vi "Teleop.vi"(10 "Match Info":T2={"Autonomous Elapsed Seconds"=0.0, "TeleOp Elapsed Seconds"=18.704, "Disabled Elapsed Seconds"=49.24, "Visited Autonomous"=FALSE, "Visited TeleOp"=TRUE, "Visited Disabled"=TRUE, "Autonomous Settings"={"Autonomous Style"=enum."Independent", "VI Refnum"=refnum}}, 11 "Call Context":T3=enum."Execute") -> ()   [LabVIEW 2015]
doc: "This VI is called for each TeleOp packet received from the DS where the robot is not disabled. It is often used to read from the joysticks and update I/O or to update setpoints for timed control loops. It should complete and return within 20 milliseconds or it may miss DS packets."
uses:
  <vilib>/Rock Robotics/WPI/DriverStation/WPI_DriverStationDerivedRobotMode.ctl
  <vilib>/Rock Robotics/WPI/DriverStation/WPI_DriverStationMatch Info.ctl
  shooter/shooter.lvclass/shooter.ctl
  intake/intake.lvclass/intake.ctl
  <vilib>/Rock Robotics/Network Tables/NT Read Boolean.vi
  <vilib>/Rock Robotics/Network Tables/NT Read Number.vi
  <vilib>/Rock Robotics/WPI/Utilities/WPI_GetSetVariantRefNum.vi
  Robot Global Data.vi
  <vilib>/Rock Robotics/Network Tables/NT Write Boolean.vi
  <vilib>/Rock Robotics/WPI/RobotDrive/WPI_RobotDriveArcadeDrive_Standard(NoSaturation).vi
  <vilib>/addons/control/pid/pid.llb/PID (DBL).vi
  <vilib>/Rock Robotics/Network Tables/NT Write Number.vi
  <vilib>/addons/control/pid/NI_PID_pid.lvlib
  <vilib>/addons/control/pid/pid.llb/PID Output Rate Limiter (DBL).vi
  shooter/shooter.lvclass
  intake/intake.lvclass
panel:
  out "Waveform Chart":cluster{dbl, dbl}(graph)={-0.002641071322889855, -0.1}
  in  "PID gains":T1={"proportional gain (Kc)"=1.0, "integral time (Ti, min)"=0.01, "derivative time (Td, min)"=0.0} {"derivative time (Td, min)" format="%.3f"; "integral time (Ti, min)" format="%.3f"; "proportional gain (Kc)" format="%.3f"}
  out "Sample Slider 0":dbl(slide) scale=0.0..5.0
  out "Sample Boolean 0":bool
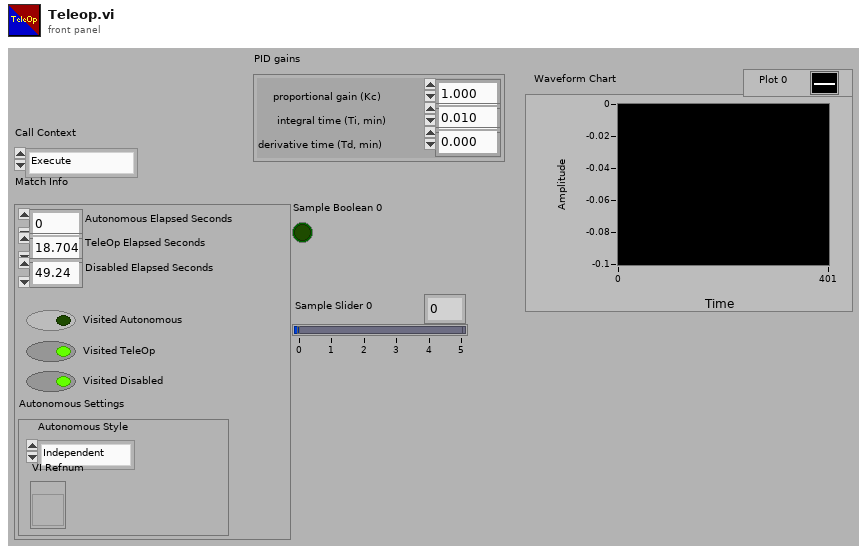
[diagram p1: front panel]
types:
  T1 = cluster{"proportional gain (Kc)":dbl, "integral time (Ti, min)":dbl, "derivative time (Td, min)":dbl}
  T2 = typedef "WPI_DriverStationMatch Info.ctl" = cluster{"Autonomous Elapsed Seconds":dbl, "TeleOp Elapsed Seconds":dbl, "Disabled Elapsed Seconds":dbl, "Visited Autonomous":bool, "Visited TeleOp":bool, "Visited Disabled":bool, "Autonomous Settings":cluster{"Autonomous Style":enum16{"Iterative", "Independent"}, "VI Refnum":refnum<vi>}}
  T3 = typedef "WPI_DriverStationDerivedRobotMode.ctl" = enum16{"Init", "Execute", "Stop"}
  T4 = typedef "WPI_JoystickDevRef.ctl" = cluster{"Device":T5}
  T5 = typedef "WPI_JoystickDeviceEnum.ctl" = enum16{"USB 0", "USB 1", "USB 2", "USB 3", "USB 4", "USB 5"}
  T6 = typedef "WPI_MotorControlDeviceRef.ctl" = cluster{"DeviceStatus":errorcluster, "Type":T7, "PWM":cluster{"PWM Channel":T8, "DeadBand":T9}, "CAN":cluster{"Device Number":u8, "Control Mode":T10, "Semaphore":T11, "Max Vout":dbl, "TalonSRX Control Mode":T12}, "Invert":bool}
  T7 = typedef "WPI_MotorControlType.ctl" = enum16{"PWM", "CAN", "CANTalonSRX"}
  T8 = typedef "FPGA_DIOPWMChannel.ctl" = enum8{"PWM 0", "PWM 1", "PWM 2", "PWM 3", "PWM 4", "PWM 5", "PWM 6", "PWM 7", "PWM 8", "PWM 9", "PWM MXP 0", "PWM MXP 1", "PWM MXP 2", "PWM MXP 3", "PWM MXP 4", "PWM MXP 5", "PWM MXP 6", "PWM MXP 7", "PWM MXP 8", "PWM MXP 9", "Invalid"}
  T9 = typedef "WPI_PWMDeadband.ctl" = cluster{"Name":string, "maxPositivePwm":i32, "minPositivePwm":i32, "centerPwm":i32, "maxNegativePwm":i32, "minNegativePwm":i32, "angularRange":u16}
  T10 = typedef "WPI_CANJaguar_ControlMode.ctl" = enum8{"Percent VBus", "Current", "Speed", "Position", "Voltage"}
  T11 = typedef "Semaphore RefNum" = refnum<k1>
  T12 = typedef "WPI_CANTalonSRX_APIControlMode.ctl" = enum8{"Percent VBus", "Speed", "Position", "Slave", "Unchanged / Invalid", "Voltage Compensation", "Current", "Motion Profile"}
  T13 = typedef "WPI_RobotDriveDevRef.ctl" = cluster{"DevStatus":errorcluster, "Motors[]":T6[], "Square Inputs":bool, "Max Output":dbl}
  T14 = typedef "WPI_SwitchDevRef.ctl" = cluster{"DevStatus":errorcluster, "DIO Channel":T15, "CntIndex":T16, "Normally Closed":bool}
  T15 = typedef "FPGA_DIOChannel.ctl" = enum8{"DIO 0", "DIO 1", "DIO 2", "DIO 3", "DIO 4", "DIO 5", "DIO 6", "DIO 7", "DIO 8", "DIO 9", "DIO MXP 0", "DIO MXP 1", "DIO MXP 2", "DIO MXP 3", "DIO MXP 4", "DIO MXP 5", "DIO MXP 6", "DIO MXP 7", "DIO MXP 8", "DIO MXP 9", "DIO MXP 10", "DIO MXP 11", "DIO MXP 12", "DIO MXP 13", "DIO MXP 14", "DIO MXP 15", "Invalid"}
  T16 = typedef "FPGA_CounterCtrSystemIndex.ctl" = enum8{"Ctr 0", "Ctr 1", "Ctr 2", "Ctr 3", "Ctr 4", "Ctr 5", "Ctr 6", "Ctr 7", "Invalid"}
  T17 = typedef "WPI_PotentiometerDevRef.ctl" = cluster{"DevStatus":errorcluster, "Analog Channel":T18, "Invert Output":bool}
  T18 = typedef "FPGA_AIChannel.ctl" = enum8{"AI 0", "AI 1", "AI 2", "AI 3", "AI MXP 0", "AI MXP 1", "AI MXP 2", "AI MXP 3", "Invalid"}
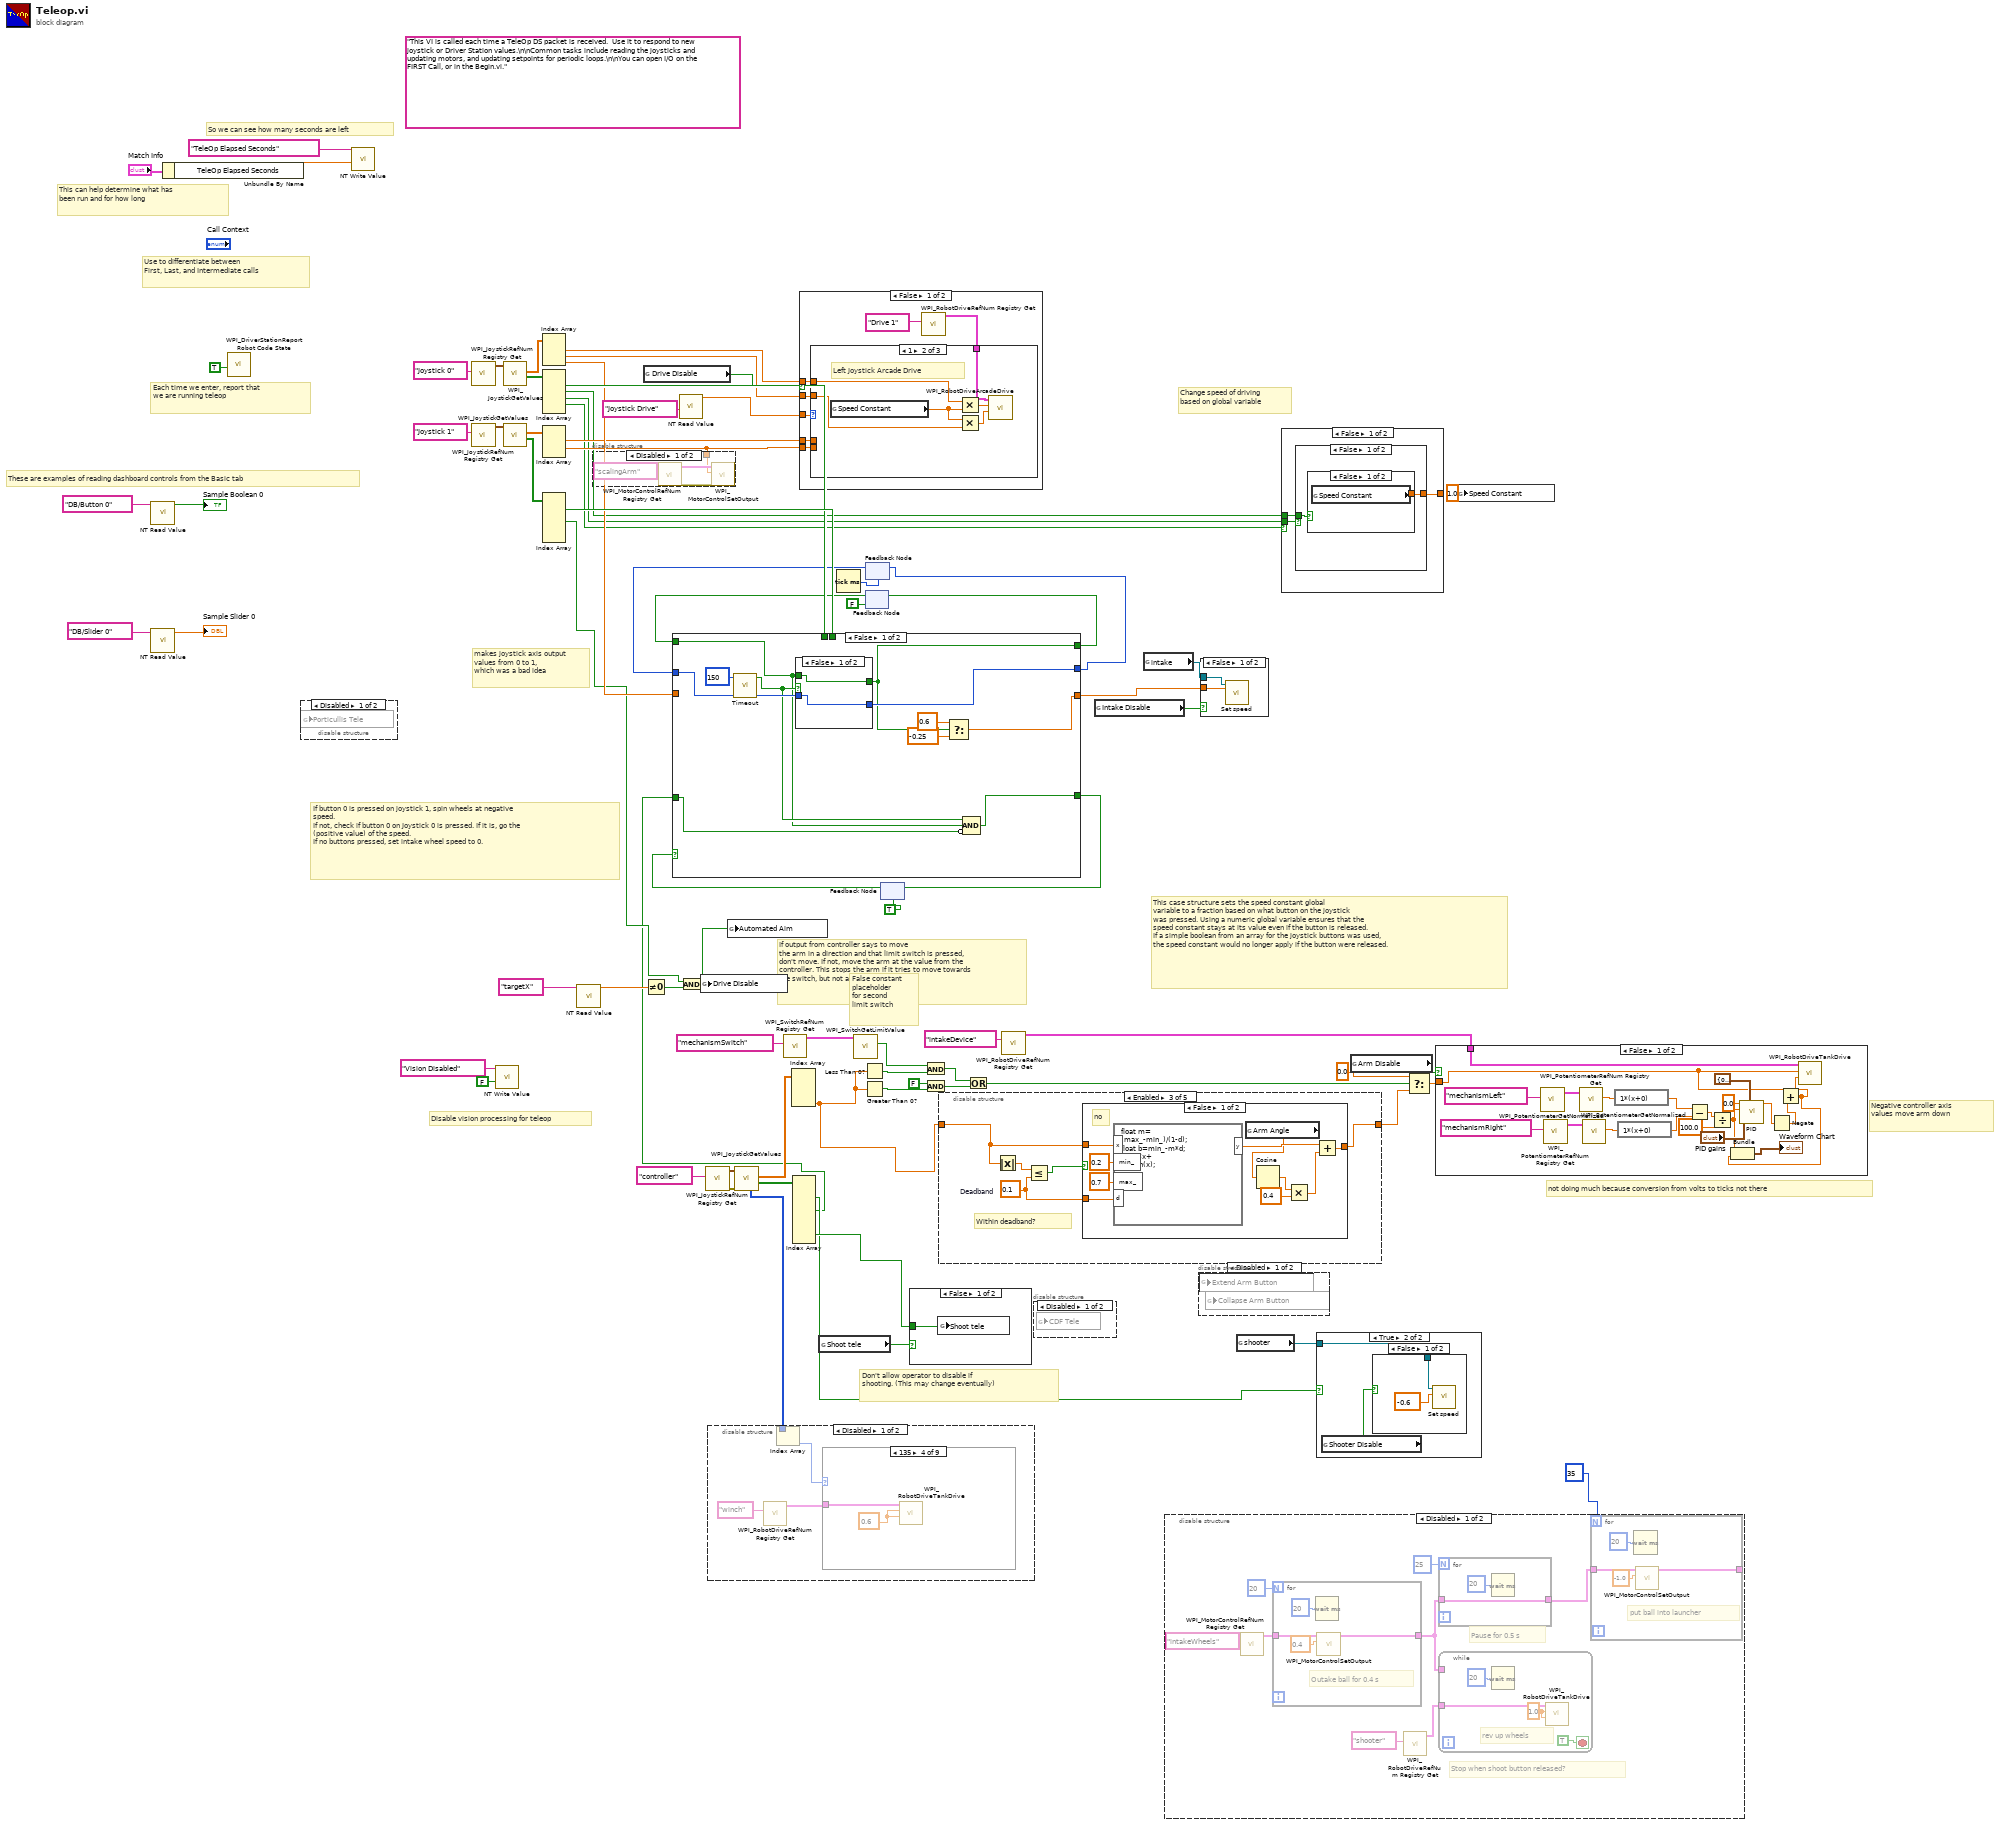
[diagram p0: block diagram]
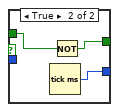
[diagram p4: hidden frame]
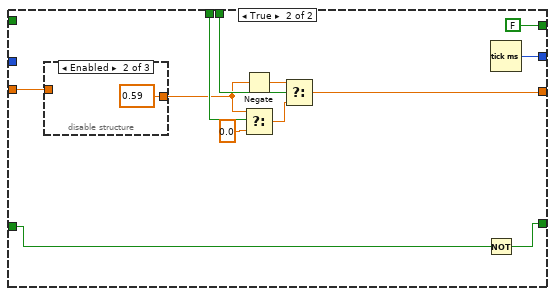
[diagram p5: hidden frame]
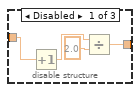
[diagram p6: hidden frame]
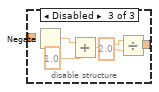
[diagram p7: hidden frame]
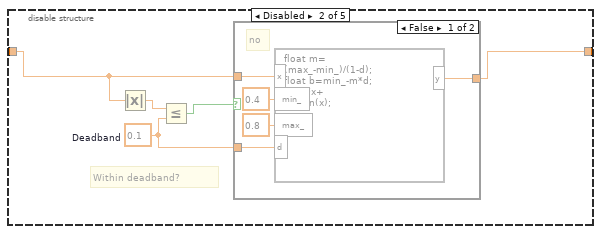
[diagram p13: hidden frame]
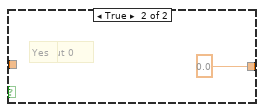
[diagram p14: hidden frame]
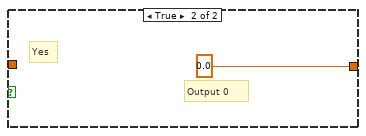
[diagram p15: hidden frame]
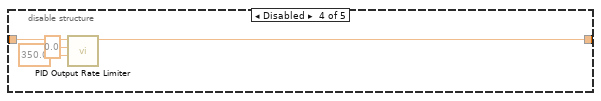
[diagram p16: hidden frame]
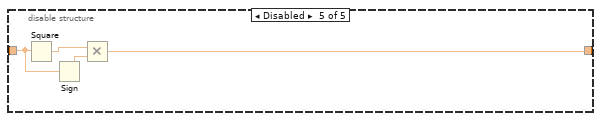
[diagram p17: hidden frame]
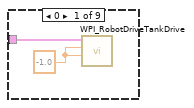
[diagram p18: hidden frame]
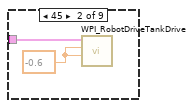
[diagram p19: hidden frame]
diagram:
  (unwired) "This VI is called each time a TeleOp DS packet is received.  Use it to respond to new joystick or Driver Station values.\n\nCommon tasks include reading the joysticks and updating motors, and updating setpoints for periodic loops.\n\nYou can open I/O on the FIRST Call, or in the Begin.vi."
  # "Don't allow operator to disable if\nshooting. (This may change eventually)"
  # "not doing much because conversion from volts to ticks not there"
  # "So we can see how many seconds are left"
  # "makes joystick axis output\nvalues from 0 to 1,\nwhich was a bad idea"
  # "If output from controller says to move \nthe arm in a direction and that limit switch is pressed,\ndon't move. If not, move the arm at the value from the\ncontroller. This stops the arm if it tries to move towards\nthe switch, but not away."
  # "False constant \nplaceholder\nfor second \nlimit switch"
  # "Disable vision processing for teleop"
  # "Change speed of driving\nbased on global variable"
  # "If button 0 is pressed on joystick 1, spin wheels at negative\nspeed.\nIf not, check if button 0 on Joystick 0 is pressed. If it is, go the\n(positive value) of the speed.\nIf no buttons pressed, set intake wheel speed to 0."
  # "Negative controller axis\nvalues move arm down"
  # "This case structure sets the speed constant global\nvariable to a fraction based on what button on the joystick\nwas pressed. Using a numeric global variable ensures that the\nspeed constant stays at its value even if the button is released.\nIf a simple boolean from an array for the joystick buttons was used,\nthe speed constant would no longer apply if the button were released."
  # "These are examples of reading dashboard controls from the Basic tab"
  # "Each time we enter, report that\nwe are running teleop"
  # "Use to differentiate between\nFirst, Last, and Intermediate calls"
  # "This can help determine what has\nbeen run and for how long"
  n1 = call-poly <vilib>:"NT Read Value.vi"("Name"="DB/Button 0" ("refnum name")) -> ("Boolean"=→"Sample Boolean 0":bool)  [unwired: 9 in, 1 out]
  n2 = call-poly <vilib>:"NT Read Value.vi"("Name"="DB/Slider 0" ("refnum name")) -> ("Numeric"=→"Sample Slider 0":dbl)  [unwired: 9 in, 1 out]
  n3 = Unbundle By Name("Match Info") -> ("TeleOp Elapsed Seconds"=w60:dbl)
  n4 = call <vilib>:"WPI_DriverStationReport Robot Code State.vi"("TeleOp"=TRUE ("Autonomous")) -> ()  [unwired: 10 in, 1 out]
  n5 = disable-structure shown="Disabled" {
    frame Disabled {
      n6 = global read "Robot Global Data.vi" "Porticullis Tele"() -> ()  [unwired: 1 in]
    }
    frame Enabled {
    }
  }
  n7 = call-poly <vilib>:"NT Write Value.vi"("Numeric"=w60, "Name"="TeleOp Elapsed Seconds") -> ()  [unwired: 9 in, 1 out]
  n8 = call <vilib>:"WPI_JoystickRefNum Registry Get.vi"("refnum name"="Joystick 0") -> ("JoystickDevRef"=w57:T4)  [unwired: 9 in, 1 out]
  n9 = call <vilib>:"WPI_JoystickRefNum Registry Get.vi"("refnum name"="Joystick 1") -> ("JoystickDevRef"=w54:T4)  [unwired: 9 in, 1 out]
  n10 = call-poly <vilib>:"NT Write Value.vi"("Boolean"=FALSE, "Name"="Vision Disabled") -> ()  [unwired: 9 in, 1 out]
  n11 = call <vilib>:"WPI_JoystickGetValues.vi"("JoystickDevRef"=w57) -> ("Buttons"=w41:bool[], "Axes"=w56:dbl[])  [unwired: 6 in, 3 out]
  n12 = call <vilib>:"WPI_JoystickGetValues.vi"("JoystickDevRef"=w54) -> ("Buttons"=w52:bool[], "Axes"=w53:dbl[])  [unwired: 6 in, 3 out]
  n13 = Index Array(array=w56) -> (element #1=w36:dbl, element #2=w39:dbl, element #3=w45:dbl)  [unwired: 3 in]
  n14 = Index Array(array=w41) -> (element #1=w50:bool, element #2=w22:bool, element #3=w6:bool, element #4=w21:bool)  [unwired: 5 in, 1 out]
  n15 = Index Array(array=w53) -> (element #1=w35:dbl, element #2=w32:dbl)  [unwired: 3 in, 1 out]
  n16 = Index Array(array=w52) -> (element #1=w51:bool, element #3=w17:bool)  [unwired: 6 in, 4 out]
  n17 = call-poly <vilib>:"NT Read Value.vi"("Name"="targetX") -> ("Numeric"=w19:dbl)  [unwired: 9 in, 1 out]
  n18 = disable-structure shown="Disabled" {
    disable-tunnel: w32 -> [w78 _]
    frame Disabled {
      n19 = call <vilib>:"WPI_MotorControlRefNum Registry Get.vi"("refnum name"="scalingArm") -> ("error out"=w80:errorcluster, "MotorControlDevRef"=w81:T6)  [unwired: 9 in]
      n20 = call <vilib>:"WPI_MotorControlSetOutput.vi"("error in (no error)"=w80, "Output"=w78, "MotorControlDevRef"=w81) -> ()  [unwired: 6 in, 3 out]
    }
    frame Enabled {
    }
  }
  n21 = global read "Robot Global Data.vi" "Drive Disable"() -> (w34:bool)
  n22 = Not Equal To 0?(x=w19) -> (x != 0?=w18:bool)
  n23 = call-poly <vilib>:"NT Read Value.vi"("Name"="Joystick Drive") -> ("Numeric"=w37:dbl)  [unwired: 9 in, 1 out]
  n24 = And(x=w17, y=w18) -> (x .and. y?=w16:bool)
  n25 = global write "Robot Global Data.vi" "Drive Disable"(w16) -> ()
  n26 = call <vilib>:"WPI_JoystickRefNum Registry Get.vi"("refnum name"="controller") -> ("error out"=w70:errorcluster, "JoystickDevRef"=w69:T4)  [unwired: 9 in]
  n27 = global write "Robot Global Data.vi" "Automated Aim"(w16) -> ()
  n28 = call <vilib>:"WPI_JoystickGetValues.vi"("error in (no error)"=w70, "JoystickDevRef"=w69) -> ("Buttons"=w71:bool[], "Axes"=w67:dbl[], "POVs"=w33:i16[])  [unwired: 5 in, 2 out]
  n29 = disable-structure shown="Disabled" {
    disable-tunnel: w33 -> [w85 _]
    frame Disabled {
      n30 = call <vilib>:"WPI_RobotDriveRefNum Registry Get.vi"("refnum name"="winch") -> ("RobotDriveDevRef"=w82:T13)  [unwired: 9 in, 1 out]
      n31 = Index Array(array=w85) -> (element=w84:i16)  [unwired: 1 in]
      n32 = case shown="135" w84 {
        tunnel: w82 -> [w87 w89 _ w90 w93 w94 _ w96 _]
        frame 0 {
          w86 = -1.0 ("Left axis value")
          n33 = call <vilib>:"WPI_RobotDriveTankDrive.vi"("Right axis value"=w86, "Left axis value"=w86, "RobotDriveDevRef"=w87) -> ()  [unwired: 6 in, 3 out]
        }
        frame 45 {
          w88 = -0.6 ("Left axis value")
          n34 = call <vilib>:"WPI_RobotDriveTankDrive.vi"("Right axis value"=w88, "Left axis value"=w88, "RobotDriveDevRef"=w89) -> ()  [unwired: 6 in, 3 out]
        }
        frame 90 {
        }
        frame 135 {
          w91 = 0.6 ("Left axis value")
          n35 = call <vilib>:"WPI_RobotDriveTankDrive.vi"("Right axis value"=w91, "Left axis value"=w91, "RobotDriveDevRef"=w90) -> ()  [unwired: 6 in, 3 out]
        }
        frame 180 {
          w92 = 1.0 ("Left axis value")
          n36 = call <vilib>:"WPI_RobotDriveTankDrive.vi"("Right axis value"=w92, "Left axis value"=w92, "RobotDriveDevRef"=w93) -> ()  [unwired: 6 in, 3 out]
        }
        frame 225 {
          w95 = -0.6 ("Left axis value")
          n37 = call <vilib>:"WPI_RobotDriveTankDrive.vi"("Right axis value"=w95, "Left axis value"=w95, "RobotDriveDevRef"=w94) -> ()  [unwired: 6 in, 3 out]
        }
        frame 270 {
        }
        frame 315 {
          w97 = -1.0 ("Left axis value")
          n38 = call <vilib>:"WPI_RobotDriveTankDrive.vi"("Right axis value"=w97, "Left axis value"=w97, "RobotDriveDevRef"=w96) -> ()  [unwired: 6 in, 3 out]
        }
        frame -1, Default {
        }
      }
    }
    frame Enabled {
    }
  }
  n39 = call <vilib>:"WPI_SwitchRefNum Registry Get.vi"("refnum name"="mechanismSwitch") -> ("SwitchDevRef"=w63:T14)  [unwired: 9 in, 1 out]
  n40 = Index Array(array=w67) -> (element #4=w23:dbl)  [unwired: 4 in, 3 out]
  n41 = Index Array(array=w71) -> (element #2=w4:bool, element #4=w3:bool, element #8=w28:bool)  [unwired: 9 in, 6 out]
  n42 = case shown="False" w34 {
    tunnel: w39 -> [w103 _]
    tunnel: w32 -> [w102 _]
    tunnel: w37 -> [w100 _]
    tunnel: w36 -> [w99 _]
    tunnel: w35 -> [w98 _]
    frame False {
      n43 = call <vilib>:"WPI_RobotDriveRefNum Registry Get.vi"("refnum name"="Drive 1") -> ("RobotDriveDevRef"=w101:T13)  [unwired: 9 in, 1 out]
      n44 = case shown="1" w100 {
        tunnel: w103 -> [w107 w112 _]
        tunnel: w102 -> [w106 _ w118]
        tunnel: w101 -> [w105 w113 w117]
        tunnel: w99 -> [_ w111 _]
        tunnel: w98 -> [_ _ w119]
        frame 0, Default {
          # "Both Joysticks Tank Drive"
          n45 = global read "Robot Global Data.vi" "Speed Constant"() -> (w108:dbl)
          n46 = Multiply(x=w107, y=w108) -> (x*y=w109:dbl)
          n47 = Multiply(x=w108, y=w106) -> (x*y=w110:dbl)
          n48 = call <vilib>:"WPI_RobotDriveTankDrive.vi"("Right axis value"=w110, "Left axis value"=w109, "RobotDriveDevRef"=w105) -> ()  [unwired: 6 in, 3 out]
        }
        frame 1 {
          # "Left Joystick Arcade Drive"
          n49 = global read "Robot Global Data.vi" "Speed Constant"() -> (w116:dbl)
          n50 = Multiply(x=w111, y=w116) -> (x*y=w115:dbl)
          n51 = Multiply(x=w116, y=w112) -> (x*y=w114:dbl)
          n52 = call-poly <vilib>:"WPI_RobotDriveArcadeDrive.vi"("Y axis value"=w114, "X axis value"=w115, "RobotDriveDevRef"=w113) -> ()  [unwired: 6 in, 3 out]
        }
        frame 2 {
          # "Right Joystick Arcade Drive"
          n53 = global read "Robot Global Data.vi" "Speed Constant"() -> (w122:dbl)
          n54 = Multiply(x=w119, y=w122) -> (x*y=w121:dbl)
          n55 = Multiply(x=w122, y=w118) -> (x*y=w120:dbl)
          n56 = call-poly <vilib>:"WPI_RobotDriveArcadeDrive.vi"("Y axis value"=w120, "X axis value"=w121, "RobotDriveDevRef"=w117) -> ()  [unwired: 6 in, 3 out]
        }
      }
    }
    frame True {
      # "Drive motors are controlled by\nloop in periodic tasks"
    }
  }
  n57 = global read "Robot Global Data.vi" "Shoot tele"() -> (w29:bool)
  n58 = Tick Count (ms)() -> (millisecond timer value=w7:u32)
  n59 = call <vilib>:"WPI_SwitchGetLimitValue.vi"("SwitchDevRef"=w63) -> ("Switch Pressed"=w62:bool)  [unwired: 8 in, 2 out]
  n60 = Less Than 0?(x=w23) -> (x < 0?=w61:bool)
  n61 = Greater Than 0?(x=w23) -> (x > 0?=w49:bool)
  n62 = feedback #1(FALSE ("Intake Disable")) -> (w11:bool)
  n63 = feedback #2(w7) -> (w8:u32)
  n64 = feedback #3(TRUE ("Intake Disable")) -> (w13:bool)
  n65 = case shown="False" w13 {
    tunnel: w51 -> [_ w149]
    tunnel: w50 -> [_ w148]
    tunnel: w45 -> [_ w146]
    tunnel: [w125 w144] -> w26
    tunnel: [w126 FALSE ("Intake Disable")] -> w12
    tunnel: w11 -> [w129 _]
    tunnel: [w131 w142] -> w9
    tunnel: w8 -> [w133 _]
    tunnel: [w127 w140] -> w5
    tunnel: w3 -> [w128 w141]
    frame False {
      n66 = call "Timeout.vi"("Start Time In"=w133, "Time Limit"=u32 150) -> ("Start Time Out"=w132:u32, "Timeout"=w130:bool)  [unwired: 8 in]
      n67 = case shown="False" w130 {
        tunnel: w132 -> [w136 _]
        tunnel: [w136 w139] -> w131
        tunnel: w129 -> [w135 w138]
        tunnel: [w135 w137] -> w126
        frame False {
        }
        frame True {
          n68 = Tick Count (ms)() -> (millisecond timer value=w139:u32)
          n69 = Not(x=w138) -> (.not. x?=w137:bool)
        }
      }
      n70 = Select(t=0.6, s=w126, f=-0.25) -> (s? t:f=w125:dbl)
      n71 = Compound Arithmetic op=AND(w130, w129, invert w128) -> (w127:bool)
    }
    frame True {
      n72 = disable-structure shown="Enabled" {
        disable-tunnel: w146 -> [w155 _ _]
        disable-tunnel: [w152 0.59 w160] -> w145
        frame Disabled {
          n73 = Increment(x=w155) -> (x+1=w154:dbl)
          n74 = Divide(x=w154, y=2.0) -> (x/y=w152:dbl)
        }
        frame Enabled {
        }
        frame Disabled {
          n75 = Negate() -> (-x=w159:dbl)  [unwired: 1 in]
          n76 = Add(x=w159, y=1.0) -> (x+y=w157:dbl)
          n77 = Divide(x=w157, y=2.0) -> (x/y=w160:dbl)
        }
      }
      n78 = Negate(x=w145) -> (-x=w147:dbl)
      n79 = Select(t=w145, s=w148, f=0.0) -> (s? t:f=w150:dbl)
      n80 = Select(t=w147, s=w149, f=w150) -> (s? t:f=w144:dbl)
      n81 = Not(x=w141) -> (.not. x?=w140:bool)
      n82 = Tick Count (ms)() -> (millisecond timer value=w142:u32)
    }
  }
  n83 = feedback-in #1(w12) -> ()
  n84 = feedback-in #2(w9) -> ()
  n85 = feedback-in #3(w5) -> ()
  n86 = case shown="False" w29 {
    tunnel: w28 -> [w162 _]
    frame False {
      n87 = global write "Robot Global Data.vi" "Shoot tele"(w162) -> ()
    }
    frame True {
    }
  }
  n88 = And(x=w62, y=w61) -> (x .and. y?=w47:bool)
  n89 = And(x=FALSE, y=w49) -> (x .and. y?=w48:bool)
  n90 = disable-structure shown="Enabled" {
    disable-tunnel: [w163 w164 w175 w194 w195] -> w31
    disable-tunnel: w23 -> [w163 w165 w176 w193 w198]
    frame Disabled {
    }
    frame Disabled {
      w166 = 0.1  # Deadband
      # "Within deadband?"
      n91 = Absolute Value(x=w165) -> (abs(x)=w168:dbl)
      n92 = Less Or Equal?(x=w168, y=w166) -> (x <= y?=w167:bool)
      n93 = case shown="False" w167 {
        tunnel: [w173 0.0 ("y")] -> w164
        tunnel: w165 -> [w170 _]
        tunnel: w166 -> [w169 _]
        frame False {
          # "no"
          n94 = formula code="float m= \n(max_-min_)/(1-d);\nfloat b=min_-m*d;\ny=m*x+\nb*sign(x);"("x"=w170, "min_"=0.4 ("input variable"), "max_"=0.8 ("input variable"), "d"=w169) -> ("y"=w173:dbl)
        }
        frame True {
          # "Yes"
          # "Output 0"
        }
      }
    }
    frame Enabled {
      w177 = 0.1  # Deadband
      # "Within deadband?"
      n95 = Absolute Value(x=w176) -> (abs(x)=w179:dbl)
      n96 = Less Or Equal?(x=w179, y=w177) -> (x <= y?=w178:bool)
      n97 = case shown="False" w178 {
        tunnel: [w181 0.0 ("y")] -> w175
        tunnel: w176 -> [w187 _]
        tunnel: w177 -> [w186 _]
        frame False {
          # "no"
          n98 = formula code="float m= \n(max_-min_)/(1-d);\nfloat b=min_-m*d;\ny=m*x+\nb*sign(x);"("x"=w187, "min_"=0.2 ("input variable"), "max_"=0.7 ("input variable"), "d"=w186) -> ("y"=w183:dbl)
          n99 = global read "Robot Global Data.vi" "Arm Angle"() -> (w180:dbl)
          n100 = Cosine(x=w180) -> (cos(x)=w185:dbl)
          n101 = Multiply(x=w185, y=0.4) -> (x*y=w182:dbl)
          n102 = Add(x=w183, y=w182) -> (x+y=w181:dbl)
        }
        frame True {
          # "Yes"
          # "Output 0"
        }
      }
    }
    frame Disabled {
      n103 = call-poly <vilib>:"PID Output Rate Limiter.vi"("output rate (EGU/min)"=350.0, "initial output"=0.0, "input (controller output)"=w193) -> ("output"=w194:dbl)  [unwired: 5 in, 1 out]
    }
    frame Disabled {
      n104 = Square(x=w198) -> (x^2=w196:dbl)
      n105 = Sign(1:w198) -> (0:w197:dbl)
      n106 = Multiply(x=w196, y=w197) -> (x*y=w195:dbl)
    }
  }
  n107 = Or(x=w47, y=w48) -> (x .or. y?=w46:bool)
  n108 = call <vilib>:"WPI_RobotDriveRefNum Registry Get.vi"("refnum name"="intakeDevice") -> ("RobotDriveDevRef"=w65:T13)  [unwired: 9 in, 1 out]
  n109 = disable-structure shown="Disabled" {
    frame Disabled {
      n110 = global read "Robot Global Data.vi" "CDF Tele"() -> ()  [unwired: 1 in]
    }
    frame Enabled {
    }
  }
  n111 = global read "Robot Global Data.vi" "Intake Disable"() -> (w27:bool)
  n112 = global read "Robot Global Data.vi" "intake"() -> (w1:refnum<class "intake.lvclass">)
  n113 = disable-structure shown="Disabled" {
    disable-tunnel: 35 -> [w199 _]
    frame Disabled {
      # "Pause for 0.5 s"
      # "Stop when shoot button released?"
      n114 = call <vilib>:"WPI_MotorControlRefNum Registry Get.vi"("refnum name"="intakeWheels") -> ("MotorControlDevRef"=w206:T6)  [unwired: 9 in, 1 out]
      n115 = for {
        N: 20 -> [_]
        tunnel: w206 -> [w214]
        tunnel: [w212] -> w203
        # "Outake ball for 0.4 s"
        n116 = Wait (ms)(milliseconds to wait=u32 20) -> ()  [unwired: 1 out]
        n117 = call <vilib>:"WPI_MotorControlSetOutput.vi"("Output"=0.4 ("initial output"), "MotorControlDevRef"=w214) -> ("MotorControlDevRef"=w212:T6)  [unwired: 7 in, 2 out]
      }
      n118 = call <vilib>:"WPI_RobotDriveRefNum Registry Get.vi"("refnum name"="shooter") -> ("RobotDriveDevRef"=w201:T13)  [unwired: 9 in, 1 out]
      n119 = for {
        N: 25 -> [_]
        tunnel: w203 -> [w220]
        tunnel: [w220] -> w200
        n120 = Wait (ms)(milliseconds to wait=u32 20) -> ()  [unwired: 1 out]
      }
      n121 = while {
        tunnel: w203 -> [_]
        tunnel: w201 -> [w209]
        stop <- TRUE stop-if-true
        w208 = 1.0 ("Left axis value")
        # "rev up wheels"
        n122 = Wait (ms)(milliseconds to wait=u32 20) -> ()  [unwired: 1 out]
        n123 = call <vilib>:"WPI_RobotDriveTankDrive.vi"("Right axis value"=w208, "Left axis value"=w208, "RobotDriveDevRef"=w209) -> ()  [unwired: 6 in, 3 out]
      }
      n124 = for {
        N: w199 -> [_]
        tunnel: w200 -> [w218]
        tunnel: [w216] -> _
        # "put ball into launcher"
        n125 = Wait (ms)(milliseconds to wait=u32 20) -> ()  [unwired: 1 out]
        n126 = call <vilib>:"WPI_MotorControlSetOutput.vi"("Output"=-1.0 ("initial output"), "MotorControlDevRef"=w218) -> ("MotorControlDevRef"=w216:T6)  [unwired: 7 in, 2 out]
      }
    }
    frame Enabled {
    }
  }
  n127 = disable-structure shown="Disabled" {
    frame Disabled {
      n128 = global read "Robot Global Data.vi" "Extend Arm Button"() -> ()  [unwired: 1 in]
      n129 = global read "Robot Global Data.vi" "Collapse Arm Button"() -> ()  [unwired: 1 in]
    }
    frame Enabled {
    }
  }
  n130 = case shown="False" w27 {
    tunnel: w26 -> [w223 _]
    tunnel: w1 -> [w222 _]
    frame False {
      n131 = call "Set speed.vi"("speed"=w223, "intake in"=w222) -> ()  [unwired: 9 in, 1 out]
    }
    frame True {
    }
  }
  n132 = global read "Robot Global Data.vi" "shooter"() -> (w2:refnum<class "shooter.lvclass">)
  n133 = case shown="False" w21 {
    tunnel: [w224 0.6 ("Speed Constant")] -> _
    tunnel: w6 -> [w226 _]
    tunnel: w22 -> [w225 _]
    frame False {
      n134 = case shown="False" w226 {
        tunnel: w225 -> [w228 _]
        tunnel: [w227 0.75] -> w224
        frame False {
          n135 = case shown="False" w228 {
            tunnel: [w229 1.0] -> w227
            frame False {
              n136 = global read "Robot Global Data.vi" "Speed Constant"() -> (w229:dbl)
            }
            frame True {
            }
          }
        }
        frame True {
        }
      }
    }
    frame True {
    }
  }
  n137 = case shown="True" w4 {
    tunnel: w2 -> [_ w233]
    frame False {
    }
    frame True {
      n138 = global read "Robot Global Data.vi" "Shooter Disable"() -> (w234:bool)
      n139 = case shown="False" w234 {
        tunnel: w233 -> [w235 _]
        frame False {
          n140 = call "Set speed.vi"("speed"=-0.6 ("Right axis value"), "shooter in"=w235) -> ()  [unwired: 9 in, 1 out]
        }
        frame True {
        }
      }
    }
  }
  n141 = global read "Robot Global Data.vi" "Arm Disable"() -> (w25:bool)
  n142 = Select(t=0.0, s=w46, f=w31) -> (s? t:f=w44:dbl)
  n143 = case shown="False" w25 {
    tunnel: w65 -> [w256 _]
    tunnel: w44 -> [w238 _]
    frame False {
      n144 = call <vilib>:"WPI_PotentiometerRefNum Registry Get.vi"("refnum name"="mechanismLeft") -> ("PotDevRef"=w248:T17)  [unwired: 9 in, 1 out]
      n145 = call <vilib>:"WPI_PotentiometerRefNum Registry Get.vi"("refnum name"="mechanismRight") -> ("PotDevRef"=w249:T17)  [unwired: 9 in, 1 out]
      n146 = call <vilib>:"WPI_PotentiometerGetNormalized.vi"("PotDevRef"=w248) -> ("Normalized Value"=w247:dbl)  [unwired: 8 in, 2 out]
      n147 = call <vilib>:"WPI_PotentiometerGetNormalized.vi"("PotDevRef"=w249) -> ("Normalized Value"=w250:dbl)  [unwired: 8 in, 2 out]
      n148 = expression code="1*(x+0)"(w247) -> (w252:dbl)
      n149 = expression code="1*(x+0)"(w250) -> (w253:dbl)
      n150 = Subtract(x=w252, y=w253) -> (x-y=w245:dbl)
      n151 = Divide(x=w245, y=100.0) -> (x/y=w242:dbl)
      n152 = call-poly <vilib>:"PID.vi"("output range"=cluster{"output high":dbl, "output low":dbl} {"output high"=0.1, "output low"=-0.1}, "PID gains"="PID gains", "process variable"=w242, "setpoint"=0.0) -> ("output"=w240:dbl)  [unwired: 6 in, 1 out]
      n153 = Negate(x=w240) -> (-x=w237:dbl)
      n154 = Add(x=w238, y=w237) -> (x+y=w239:dbl)
      n155 = Bundle(w242, w239) -> (→"Waveform Chart":cluster{dbl, dbl})  [unwired: 1 in]
      n156 = call <vilib>:"WPI_RobotDriveTankDrive.vi"("Right axis value"=w239, "Left axis value"=w238, "RobotDriveDevRef"=w256) -> ()  [unwired: 6 in, 3 out]
    }
    frame True {
    }
  }
  n157 = global write "Robot Global Data.vi" "Speed Constant"(1.0 ("Speed Constant")) -> ()
